vi "konwersja_referencji_do_kontrolki.vi"(8 "error in (no error)":errorcluster, 11 "SpecyficControl":refnum<vi>[](array[refnum])) -> (0 "error out":errorcluster, 3 "ControlClas":refnum<vi>[](array[refnum]))   [LabVIEW 2013]
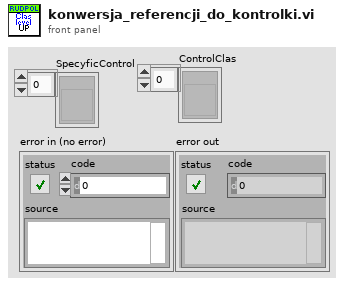
[diagram p1: front panel]
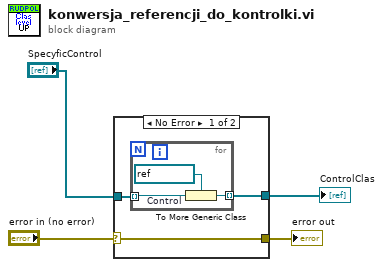
[diagram p0: block diagram]
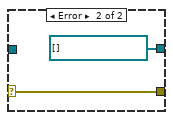
[diagram p2: hidden frame]
diagram:
  n1 = case shown="No Error" "error in (no error)" {
    selector: "error in (no error)" -> [w5 w11]
    tunnel: [w7 refnum<vi>[] []] -> w4
    tunnel: "SpecyficControl" -> [w6 _]
    tunnel: [w5 w11] -> w2
    frame No Error {
      n2 = for {
        tunnel: w6 -> [w10] mode=indexing
        tunnel: [w9] -> w7 mode=indexing
        w8 = refnum<vi> refnum  # Control
        n3 = To More Generic Class(target class=w8, reference=w10) -> (generic class reference=w9:refnum<vi>)
      }
    }
    frame Error {
    }
  }
  "ControlClas" <- w4
  "error out" <- w2
